vi "GEvt-Filter Global Log - v1.2.vi"(6 "Level (Normal)":T1, 7 "Rules":T2={"Global"={"CSM"=[], "LogType"=[], "State"=[], "StateType"=[], "Broadcast"=[], "UserLog"=[]}, "CSM"={"LogType"=[], "State"=[], "StateType"=[], "Broadcast"=[], "UserLog"=[]}, "PeriodicMessageFilter"={"Enable"=TRUE, "Threshold(#/s)"=2.0, "CheckPeriod(s)"=1.0}}, 8 "Matched Previous?":bool, 11 "Cross CSM Data (In)":T5) -> (0 "Matched? (Dup)":bool, 1 "Additional Info":string[](array[string]), 3 "Cross CSM Data":T5)   [LabVIEW 2017, in "Communicable State Machine.lvlib"]
uses:
  Communicable State Machine.lvlib
  Typedef/_CSM_GlobalLog_MSG.ctl
  Typedef/_CSM_Response Source Message.ctl
  Typedef/_CSM_GlobalLog_MSG_TYPE.ctl
  Typedef/_CSM_GlobalLog Filter Rules - v1.2.ctl
  Typedef/_CSM_GlobalLog_STATE_TYPE.ctl
  Utility/_support/Periodic String Filter Level.ctl
  LogFilter/SettingVIs/Set Periodic Log Filter.vi
  LogFilter/SettingVIs/Set CSM UserLog Filter.vi
  LogFilter/SettingVIs/Set CSM Broadcast Filter.vi
  LogFilter/SettingVIs/Set CSM StateType Filter.vi
  LogFilter/SettingVIs/Set Global StateType Filter.vi
  LogFilter/SettingVIs/Set CSM State Filter.vi
  LogFilter/SettingVIs/Set CSM LogType Filter.vi
  LogFilter/SettingVIs/Set Global UserLog Filter.vi
  LogFilter/SettingVIs/Set Global Broadcast Filter.vi
  LogFilter/SettingVIs/Set Global State Filter.vi
  LogFilter/SettingVIs/Set Global LogType Filter.vi
  LogFilter/SettingVIs/Set Global CSM Filter.vi
  LogFilter/LogFilter.lvclass
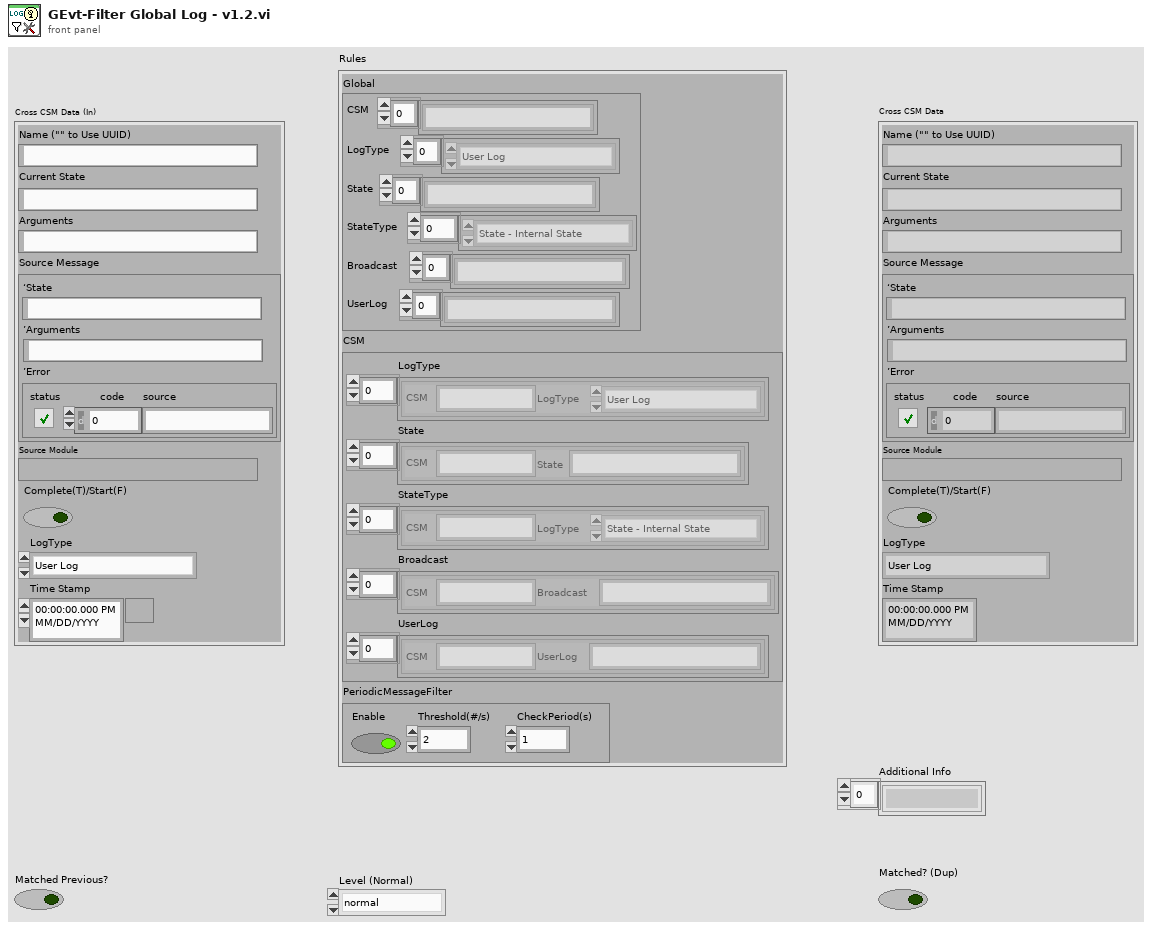
[diagram p1: front panel]
types:
  T1 = typedef "Communicable State Machine.lvlib/Periodic String Filter Level.ctl" = enum16{"normal", "L1", "L2", "L3", "L4"}
  T2 = typedef "Communicable State Machine.lvlib/_CSM_GlobalLog Filter Rules - v1.2.ctl" = cluster{"Global":cluster{"CSM":string[], "LogType":T3[], "State":string[], "StateType":T4[], "Broadcast":string[], "UserLog":string[]}, "CSM":cluster{"LogType":cluster{"CSM":string, "LogType":T3}[], "State":cluster{"CSM":string, "State":string}[], "StateType":cluster{"CSM":string, "LogType":T4}[], "Broadcast":cluster{"CSM":string, "Broadcast":string}[], "UserLog":cluster{"CSM":string, "UserLog":string}[]}, "PeriodicMessageFilter":cluster{"Enable":bool, "Threshold(#/s)":dbl, "CheckPeriod(s)":dbl}}
  T3 = typedef "Communicable State Machine.lvlib/_CSM_GlobalLog_MSG_TYPE.ctl" = enum16{"User Log", "State Change", "Status", "Interrupt", "Register", "Unregister", "Error Log", "Module Created", "Module Destroyed", "Async Message", "No-Rep Async Message", "Sync Message", "AsyncMsg Complete", "SyncMsg Complete"}
  T4 = typedef "Communicable State Machine.lvlib/_CSM_GlobalLog_STATE_TYPE.ctl" = enum16{"State - Internal State", "State - External Message", "State - Response", "State - Complete"}
  T5 = typedef "Communicable State Machine.lvlib/_CSM_GlobalLog_MSG.ctl" = cluster{"Name (\"\" to Use UUID)":string, "Current State":string, "Arguments":string, "Source Message":T6, "Source Module":string, "Complete(T)/Start(F)":bool, "LogType":T3, "Time Stamp":timestamp}
  T6 = typedef "Communicable State Machine.lvlib/_CSM_Response Source Message.ctl" = cluster{"‘State":string, "’Arguments":string, "’Error":errorcluster}
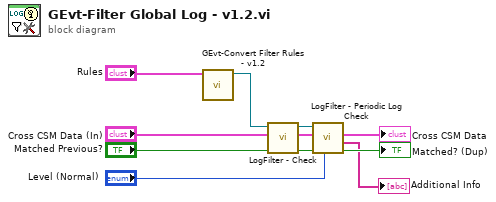
[diagram p0: block diagram]
diagram:
  n1 = call "GEvt-Convert Filter Rules - v1.2.vi"("Rules-v1.2"="Rules") -> ("GlobalLogFilter"=w10:refnum<class "LogFilter.lvclass">)  [unwired: 10 in]
  n2 = call "LogFilter - Check.vi"("Matched Previous?"="Matched Previous?", "Cross CSM Data In"="Cross CSM Data (In)", "GlobalLogFilter In"=w10) -> ("Matched? (Dup)"=w8:bool, "Cross CSM Data Out"=w4:T5, "GlobalLogFilter.lvclass (Dup)"=w5:refnum<class "LogFilter.lvclass">)  [unwired: 6 in]
  n3 = call "LogFilter - Periodic Log Check.vi"("Level (Normal)"="Level (Normal)", "Matched Previous?"=w8, "Cross CSM Data In"=w4, "GlobalLogFilter In"=w5) -> ("Matched? (Dup)"=→"Matched? (Dup)":bool, "Additional Info"=→"Additional Info":string[], "Cross CSM Data Out"=→"Cross CSM Data":T5)  [unwired: 3 in, 2 out]
